vi "robot_initial.vi"   [LabVIEW 2020]
uses:
  Robot-HL/small_scara_interface/small_scara_interface.lvlib
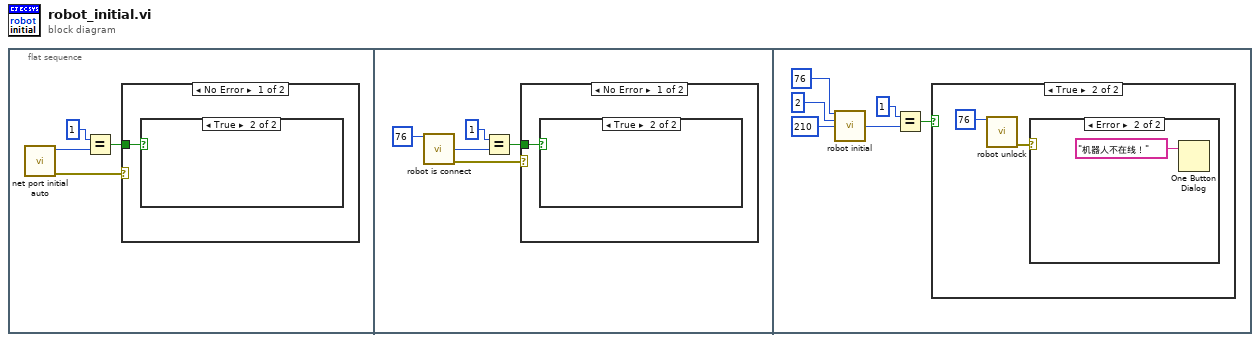
[diagram p0: block diagram]
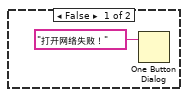
[diagram p2: hidden frame]
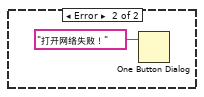
[diagram p3: hidden frame]
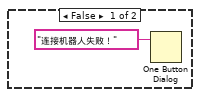
[diagram p4: hidden frame]
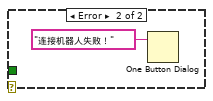
[diagram p5: hidden frame]
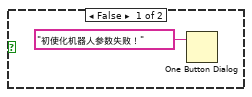
[diagram p6: hidden frame]
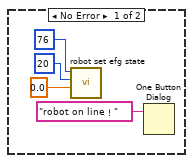
[diagram p7: hidden frame]
diagram:
  n1 = flat-sequence {
    frame #0 {
      n2 = call "net port initial auto.vi"() -> ("error out"=w2:errorcluster, "function return"=w3:i32)  [unwired: 10 in]
      n3 = Equal?(x=1, y=w3) -> (x = y?=w4:bool)
      n4 = case shown="No Error" w2 {
        tunnel: w4 -> [w5 _]
        frame No Error {
          n5 = case shown="True" w5 {
            frame False {
              n6 = One Button Dialog(message="打开网络失败！" ("消息")) -> ()  [unwired: 1 in, 1 out]
            }
            frame True {
            }
          }
        }
        frame Error {
          n7 = One Button Dialog(message="打开网络失败！" ("消息")) -> ()  [unwired: 1 in, 1 out]
        }
      }
    }
    frame #1 {
      n8 = call "robot is connect.vi"("robot_id"=76) -> ("function return"=w8:i32, "error out"=w9:errorcluster)  [unwired: 12 in, 1 out]
      n9 = Equal?(x=1, y=w8) -> (x = y?=w12:bool)
      n10 = case shown="No Error" w9 {
        tunnel: w12 -> [w13 _]
        frame No Error {
          n11 = case shown="True" w13 {
            frame False {
              n12 = One Button Dialog(message="连接机器人失败！" ("消息")) -> ()  [unwired: 1 in, 1 out]
            }
            frame True {
            }
          }
        }
        frame Error {
          n13 = One Button Dialog(message="连接机器人失败！" ("消息")) -> ()  [unwired: 1 in, 1 out]
        }
      }
    }
    frame #2 {
      n14 = call "robot initial.vi"("robot_id"=76, "generation"=2, "z_trail"=210) -> ("function return"=w19:i32)  [unwired: 10 in, 2 out]
      n15 = Equal?(x=1, y=w19) -> (x = y?=w21:bool)
      n16 = case shown="True" w21 {
        frame False {
          n17 = One Button Dialog(message="初使化机器人参数失败！" ("消息")) -> ()  [unwired: 1 in, 1 out]
        }
        frame True {
          n18 = call "robot unlock.vi"("robot_id"=76) -> ("error out"=w24:errorcluster)  [unwired: 14 in]
          n19 = case shown="Error" w24 {
            frame No Error {
              n20 = call "robot set efg state.vi"("distance"=sgl 0.0, "type"=20, "robot_id"=76) -> ()  [unwired: 8 in, 1 out]
              n21 = One Button Dialog(message="robot on line！" ("消息")) -> ()  [unwired: 1 in, 1 out]
            }
            frame Error {
              n22 = One Button Dialog(message="机器人不在线！" ("消息")) -> ()  [unwired: 1 in, 1 out]
            }
          }
        }
      }
    }
  }
